vi "Sesnor_Degree_Finder.vi"(1 "Minimum Volts":dbl, 2 "Voltage":dbl(knob) scale=0.5..4.5, 3 "Max Volts":dbl) -> (0 "Degrees":dbl)   [LabVIEW 2013]
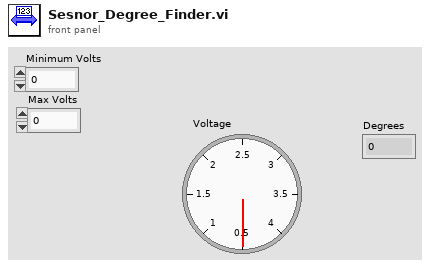
[diagram p1: front panel]
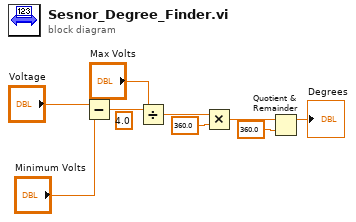
[diagram p0: block diagram]
diagram:
  (unwired) 4.0 ("y")
  n1 = Subtract(x="Voltage", y="Minimum Volts") -> (x-y=w8:dbl)
  n2 = Divide(x=w8, y="Max Volts") -> (x/y=w7:dbl)
  n3 = Multiply(x=w7, y=360.0) -> (x*y=w5:dbl)
  n4 = Quotient & Remainder(x=w5, y=360.0) -> (x-y*floor(x/y)=→"Degrees":dbl)  [unwired: 1 out]
